vi "loadOutcount1.vi"() -> ()   [LabVIEW 2012]
uses:
  Global1.vi
  <vilib>/Utility/file.llb/Read From Spreadsheet File (string).vi
  <vilib>/addons/database/Connection.llb/DB Tools Open Connec (Path).vi
  <vilib>/addons/database/Connection.llb/Conn Execute.vi
  <vilib>/addons/database/Recordset.llb/Rec Destroy - Connection.vi
  <vilib>/addons/database/NI_Database_API.lvlib
panel:
  out "appended array":string[](array[string])
  out "element":string
  out "OK":bool
  out "Output":string
  out "error out":errorcluster
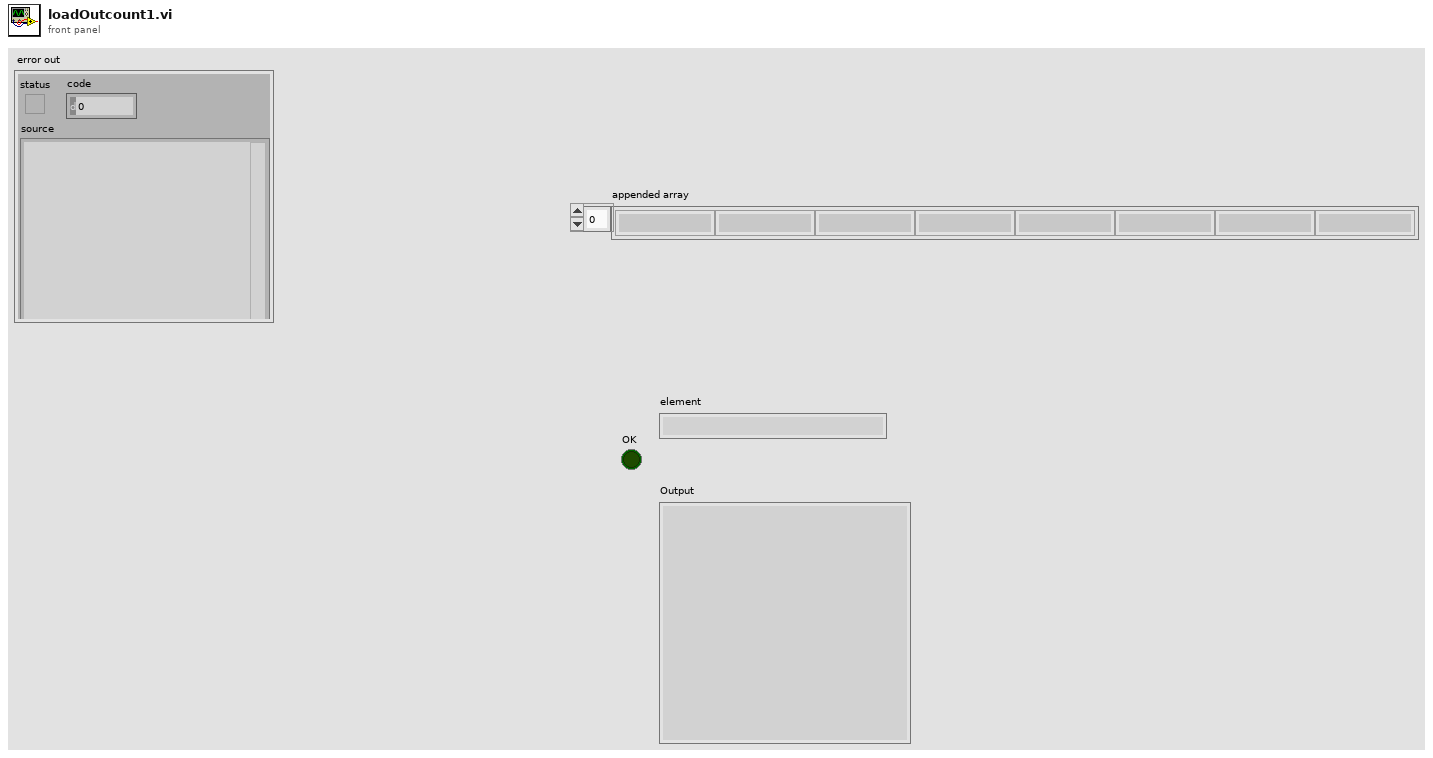
[diagram p1: front panel]
types:
  T1 = typedef "NI_Database_API.lvlib/Conn ObjectReference.ctl" = refnum<k1>
  T2 = typedef "NI_Database_API.lvlib/Rec ObjectReference.ctl" = refnum<k1>
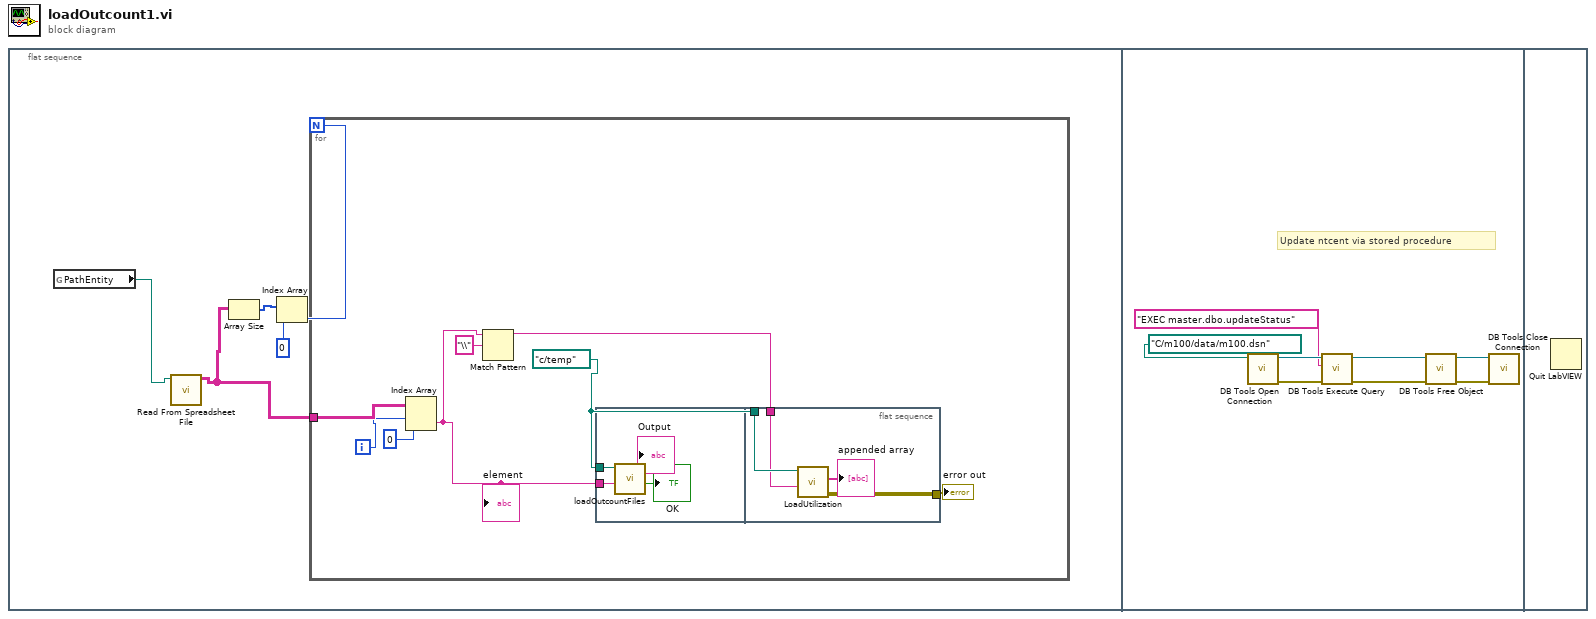
[diagram p0: block diagram]
diagram:
  n1 = flat-sequence {
    frame #0 {
      n2 = global read "Global1.vi" "PathEntity"() -> (w1:path)
      n3 = call-poly <vilib>:"Read From Spreadsheet File.vi"("file path (dialog if empty)"=w1) -> ("all rows"=w2:string[][])  [unwired: 6 in, 4 out]
      n4 = Array Size(array=w2) -> (size(s)=w5:i32[])
      n5 = Index Array(array=w5, index=0) -> (element=w3:i32)
      n6 = for {
        N: w3 -> [_]
        tunnel: w2 -> [w13]
        i -> [w11]
        w8 = path "c:/temp" ("working directory")
        n7 = Index Array(array=w13, index (row)=w11, index (col)=0 ("disabled index (col)")) -> (element=w9:string)
        "element" <- w9
        n8 = Match Pattern(string=w9, regular expression="\\") -> (before substring=w7:string)  [unwired: 1 in, 3 out]
        n9 = flat-sequence {
          tunnel: w9 -> [w17]
          tunnel: w8 -> [w16]
          tunnel: w8 -> [w21]
          tunnel: w7 -> [w20]
          tunnel: [w19] -> w6
          frame #0 {
            n10 = call "loadOutcountFiles.vi"("folder"=w17, "working directory"=w16) -> ("OK"=→"OK":bool, "Output"=→"Output":string)  [unwired: 8 in]
          }
          frame #1 {
            n11 = call "LoadUtilization.vi"("base path"=w21, "machine"=w20) -> ("appended array"=→"appended array":string[], "error out"=w19:errorcluster)  [unwired: 6 in]
          }
        }
        "error out" <- w6
      }
    }
    frame #1 {
      # "Update ntcent via stored procedure"
      n12 = call-poly <vilib>:"DB Tools Open Connection.vi"("connection information"=path "C:/m100/data/m100.dsn") -> ("error out"=w27:errorcluster, "connection reference"=w28:T1)  [unwired: 7 in]
      n13 = call-poly <vilib>:"DB Tools Execute Query.vi"("error in (no error)"=w27, "SQL query"="EXEC master.dbo.updateStatus", "connection reference"=w28) -> ("error out"=w29:errorcluster, "recordset reference"=w26:T2)  [unwired: 5 in]
      n14 = call-poly <vilib>:"DB Tools Free Object.vi"("error in (no error)"=w29, "recordset reference"=w26) -> ("error out"=w24:errorcluster, "connection reference"=w25:T1)  [unwired: 8 in]
      n15 = call <vilib>:"DB Tools Close Connection.vi"("error in (no error)"=w24, "connection reference"=w25) -> ()  [unwired: 5 in, 1 out]
    }
    frame #2 {
      n16 = Quit LabVIEW() -> ()  [unwired: 1 in]
    }
  }
